vi "Write Tx Channel Dependent Nodes.vi"(8 "error in (no error)":errorcluster, 10 "Dependent Node Refs":T1[](array[typedef]) format="%.0x", 11 "Node Ptr":T1 format="%.0x") -> (0 "error out":errorcluster, 3 "Node Ptr out":T1 format="%.0x")   [LabVIEW 2019, in "UDP-Custom-Device System Explorer.lvlib" / "Tx Channel Section Accessors.lvlib"]
uses:
  Tx Channel Section Accessors.lvlib
  <vilib>/NI VeriStand/Custom Device API/Custom Device Item Ref.ctl
  Shared/Constants.vi
  <vilib>/NI VeriStand/Custom Device Tools/Custom Device Utility Library/Custom Device Utility Library.lvlib
  Shared/UDP-Custom-Device Shared.lvlib
  <vilib>/NI VeriStand/Custom Device API/Custom Device API.lvlib
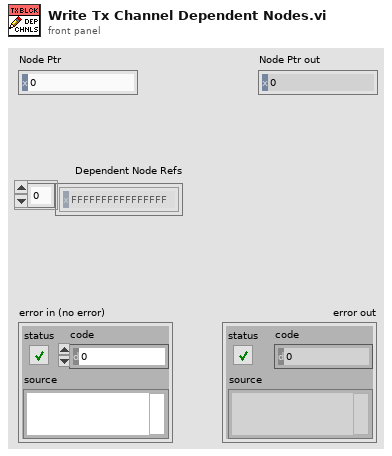
[diagram p1: front panel]
types:
  T1 = typedef "Custom Device API.lvlib/Custom Device Item Ref.ctl" = u64
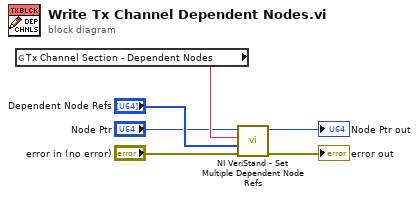
[diagram p0: block diagram]
diagram:
  n1 = global read "Constants.vi" "Tx Channel Section - Dependent Nodes"() -> (w6:string)
  n2 = call <vilib>:"NI VeriStand - Set Multiple Dependent Node Refs.vi"("error in (no error)"="error in (no error)", "Dependent Node Refs"="Dependent Node Refs", "Base Property Name"=w6, "Item Ref in"="Node Ptr") -> ("error out"=→"error out":errorcluster, "Item Ref out"=→"Node Ptr out":T1)  [unwired: 6 in]
